vi "Dashboard Main.vi"() -> ()   [LabVIEW 2013]
uses:
  <vilib>/event_ctls.llb/eventvkey.ctl
  <vilib>/Rock Robotics/WPI/Dashboard/WPI_DashboardLogging Global.vi
  <vilib>/Utility/config.llb/Write Key (String).vi
  <vilib>/Utility/config.llb/Write Key (I32).vi
  <vilib>/Utility/config.llb/NI_LVConfig.lvlib
panel:
  out "Image Message":string="Timeout in Camera Communications"
  in  "Rec Mode":enum32{"Stop", "Record", "Playback"}(radio)
  in  "Dashboard Tab":T1(tab)
  out "Pressure":dbl
  out "?":bool
  in  "?":bool
  out "Shoot":bool
  out "Rear Right Power":dbl(slide) scale=0.0..1.0
  out "Front Right Power":dbl(slide) scale=0.0..1.0
  out "Front Left Power":dbl(slide) scale=0.0..1.0
  out "Front Left Wheel":dbl(knob) scale=-3.14..3.14
  out "Front Right Wheel":dbl(knob) scale=-3.14..3.14
  out "Rear Right Wheel":dbl(knob) scale=-3.14..3.14
  in  "Camera Settings":T2={"Frame Rate"=30, "Compression"=30, "Size"=1} {"Frame Rate" scale=1.0..30.0; "Size" items=["640x480", "320x240", "160x120"]}
  out "Mode":T3(ring)=enum."Auto Disabled"
  out "Camera IP":string
  in  "DB Camera Config":bool
  out "fps":dbl format="%#.1g"
  out "Mbps":dbl format="%#.1g"
  out "Mbps 2":bool
  out "Rear Left Wheel":dbl(knob) scale=-3.14..3.14
  out "Rear Left Power":dbl(slide) scale=0.0..1.0
  in  "Slider 1":dbl(slide) scale=0.0..100.0
  in  "Autonomous Type":u16(ring) items=["One Ball", "Two Ball", "Basic"]
  in  "Test Slider":dbl(slide) scale=0.0..100.0 scale format="%#_3g"
  in  "On/Off":bool caption="Solenoid"
  in  "Test Name":u16(ring) items=["Select the test to run...", "Example Test", "-------------------------------", "List of tests is built in robot code.", "Replace with your own automated tests."]
  in  "Test Tree":string(tree)
  in  "Motor":cluster{"Value":dbl, "Enable":bool} {"Value" scale=-1.0..1.0 scale format="%#_3g"}
  out "Progress":T4 {"Test Progress" scale=0.0..100.0}
  in  "Rev/Fwd":cluster{"Forward":bool, "Reverse":bool}
  in  "Test Ring":u16(ring) items=["Auto", "Fixed indoor", "Fixed outdoor 1", "Fixed outdoor 2", "Fixed fluorescent 1", "Fixed fluorescent 2", "Hold current"]
  in  "Listbox":i32(listbox)
  out "Tree":string(tree)
  out "Camera Image":T5(plugin-control)
  in  "Enable":bool
  # "Customize by placing controls and indicators here and name to\nmatch Dashboard Variables on robot."
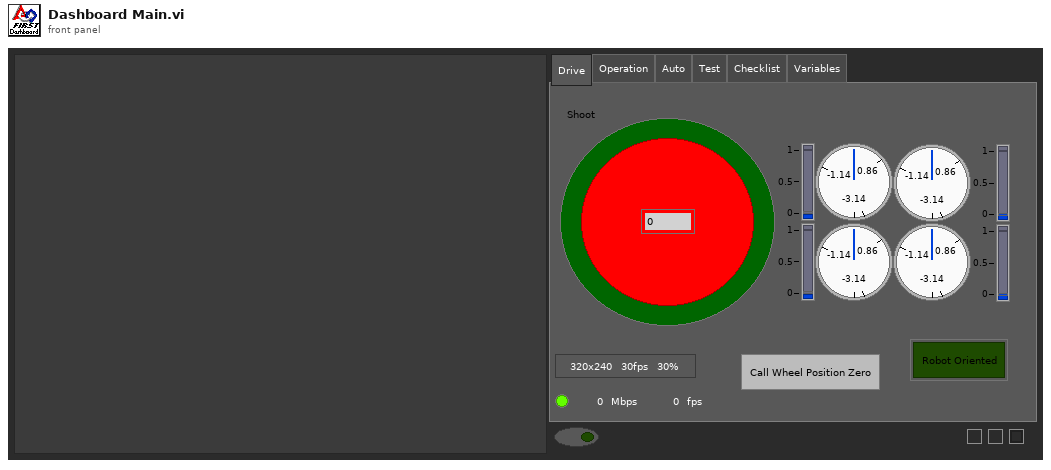
[diagram p1: front panel]
types:
  T1 = enum32{"Drive", "Operation", "Auto", "Test", "Checklist", "Variables"}
  T2 = cluster{"Frame Rate":i32, "Compression":i32, "Size":u16}
  T3 = enum8{"Tele-Op Disabled", "Tele-Op Enabled", "Auto Disabled", "Auto Enabled", "Test Disabled", "Test Enabled", ""}
  T4 = cluster{"Test Progress":u8, "Test Progress Text":string}
  T5 = typedef "IMAQ Image.ctl" = refnum<image>
  T6 = typedef "Image Type" = u32
  T7 = cluster{"Digital Inputs":bool[], "Digital Outputs":bool[]}
  T8 = cluster{"Competition mode":bool, "Robot Link":bool, "Autonomous":bool, "Enabled":bool, "E-Stop":bool, "Simulated":bool, "TestMode":bool, "Docked Window":bool}
  T9 = typedef "NI_LVConfig.lvlib/Config Data RefNum.ctl" = refnum<k1>
  T10 = typedef "eventvkey.ctl" = enum16{"ASCII", "Enter", "Return", "Shift", "Ctrl", "Alt", "Cmd", "Opt", "Caps", "NumLock", "Clear", "Break", "Up", "Down", "Left", "Right", "Insert", "Delete", "Home", "End", "PageUp", "PageDown", "Escape", "Help", "Pause", "ScrollLock", "F1", "F2", "F3", "F4", "F5", "F6", "F7", "F8", "F9", "F10", "F11", "F12", "F13", "F14", "F15", "F16", "F17", "F18", "F19", "F20", "F21", "F22", "F23", "F24", "Play", "VolumeUp", "VolumeDown", "Mute", "Two Byte Char"}
  T11 = cluster{"Image Size":bool, "Image Type":bool, "Pixel Value":bool, "ROI Information":bool, "Zoom Factor":bool}
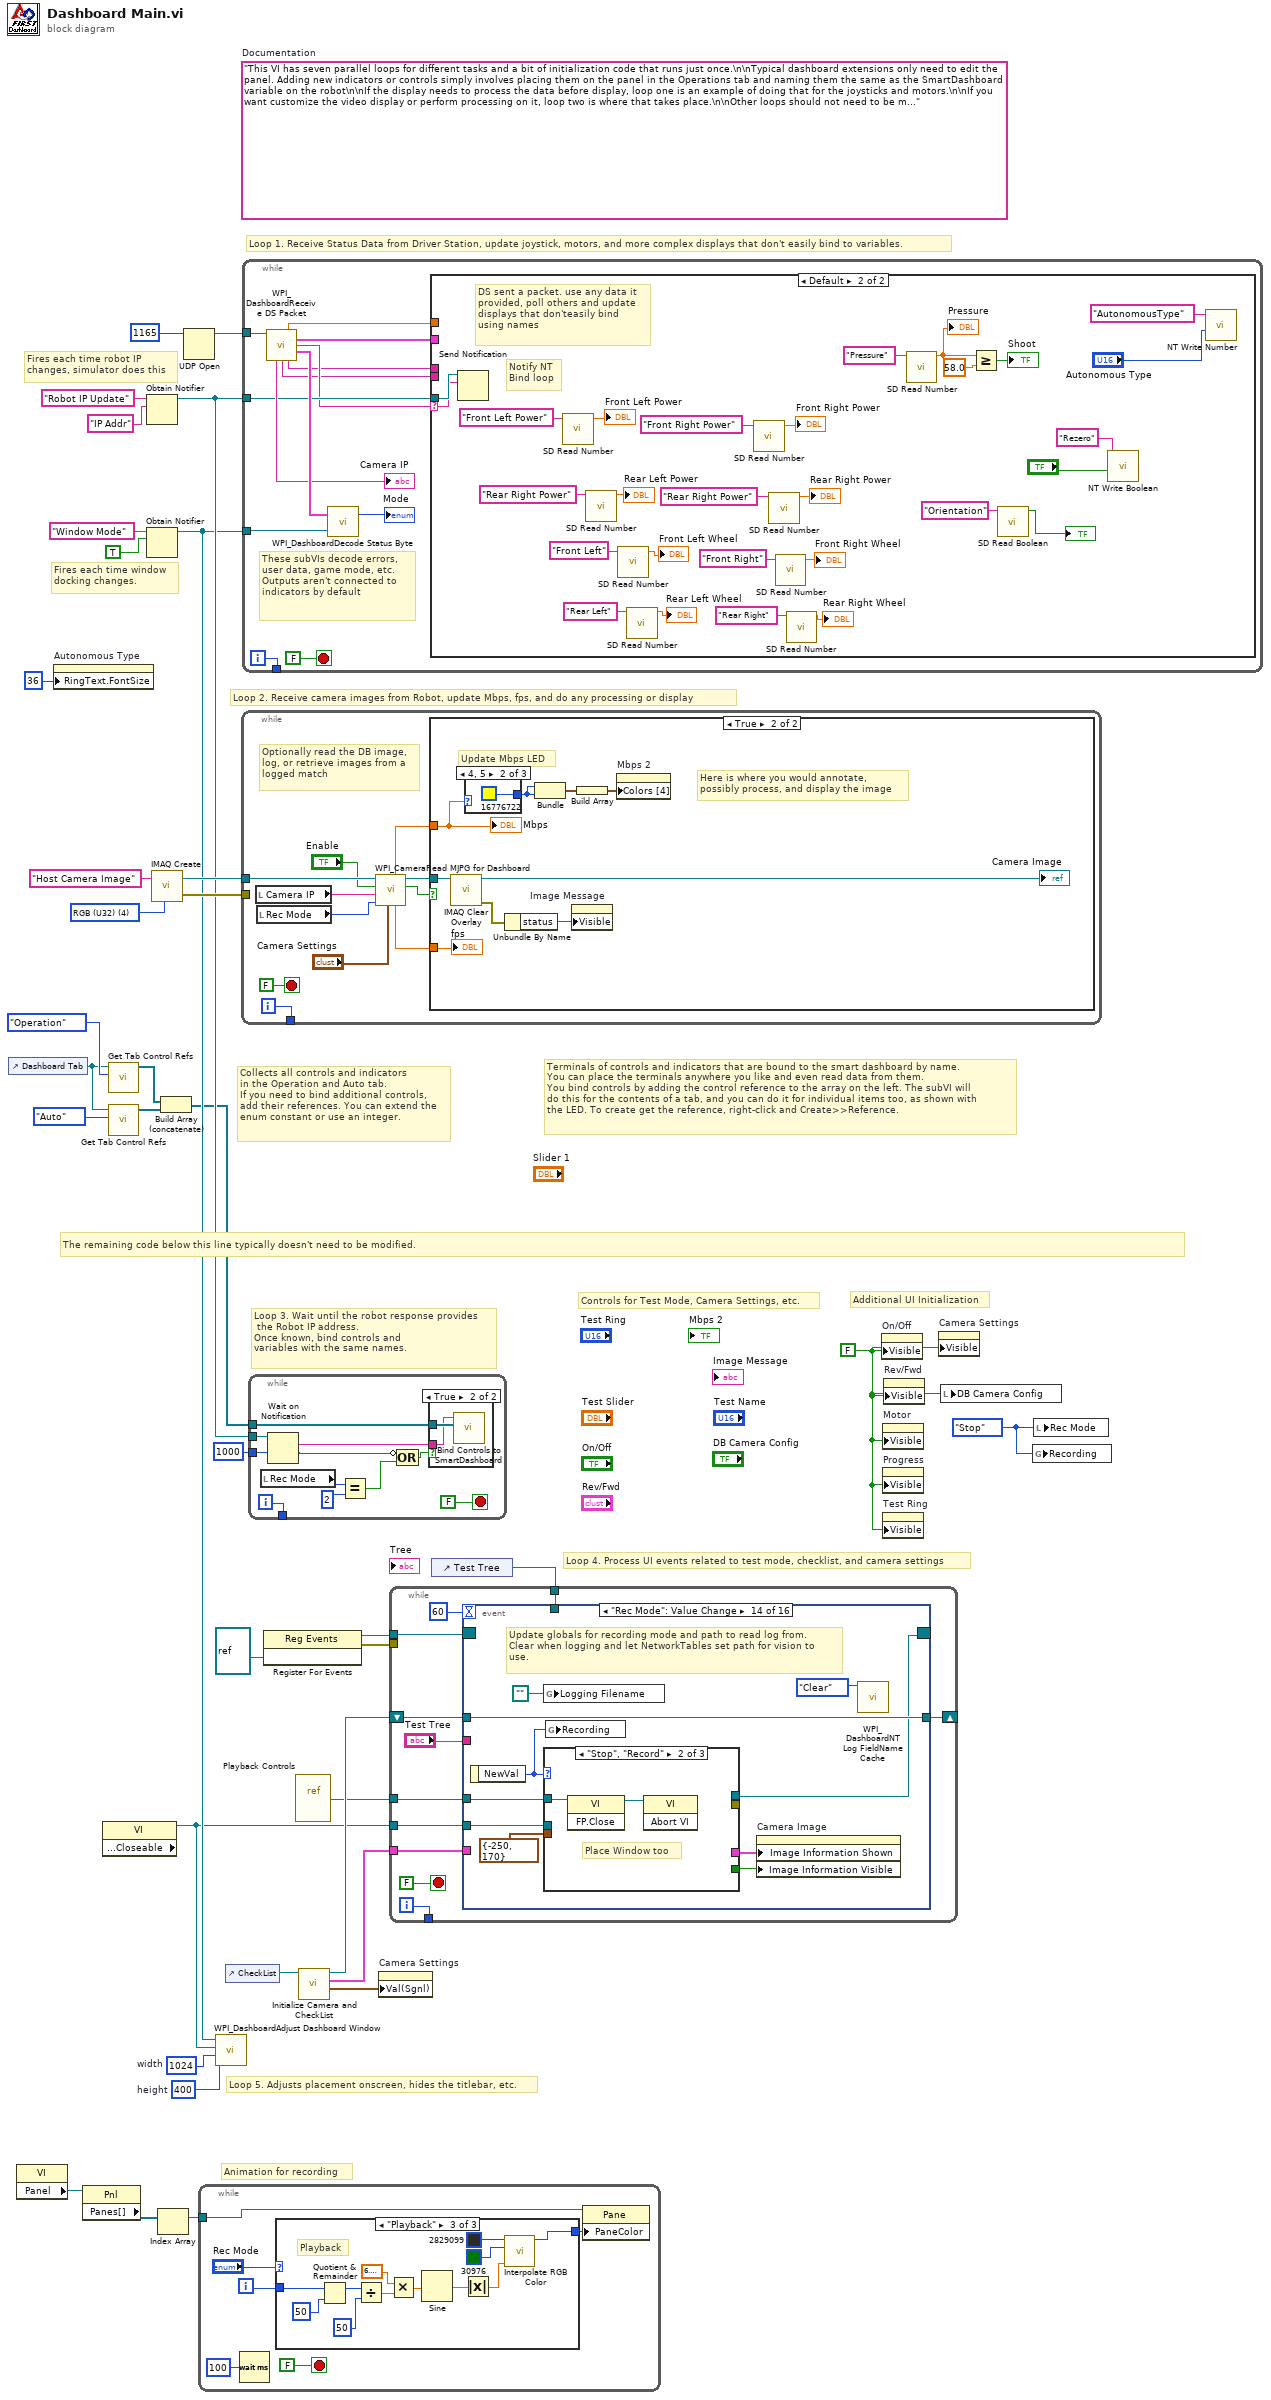
[diagram p0: block diagram]
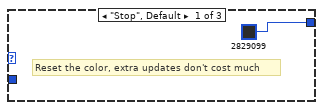
[diagram p2: hidden frame]
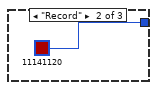
[diagram p3: hidden frame]
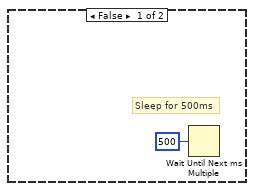
[diagram p5: hidden frame]
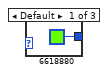
[diagram p6: hidden frame]
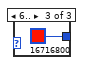
[diagram p7: hidden frame]
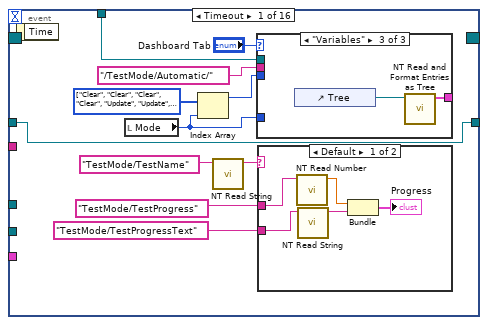
[diagram p8: hidden frame]
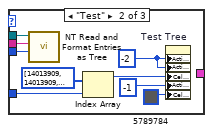
[diagram p10: hidden frame]
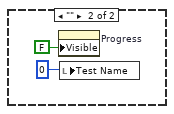
[diagram p11: hidden frame]
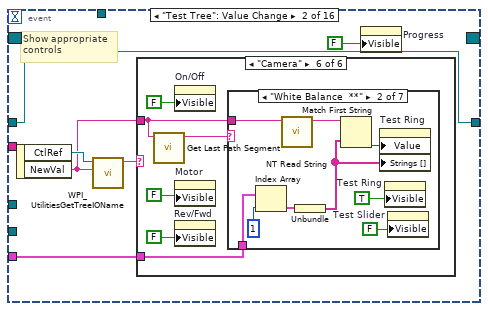
[diagram p12: hidden frame]
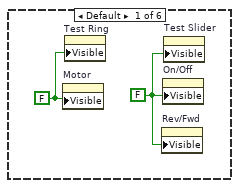
[diagram p13: hidden frame]
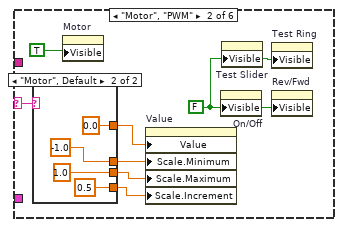
[diagram p14: hidden frame]
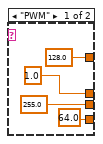
[diagram p15: hidden frame]
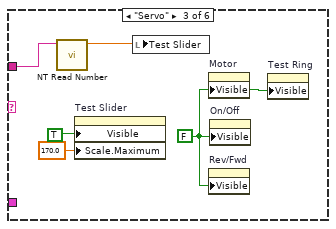
[diagram p16: hidden frame]
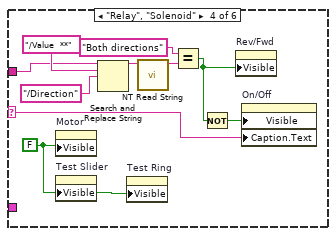
[diagram p17: hidden frame]
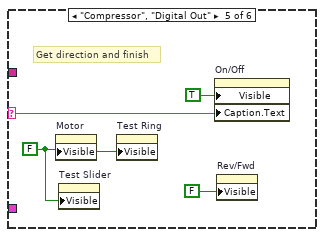
[diagram p18: hidden frame]
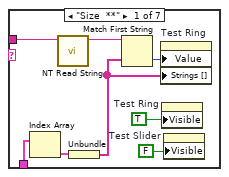
[diagram p19: hidden frame]
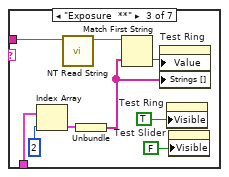
[diagram p20: hidden frame]
diagram:
  w8 = enum32{"Stop", "Record", "Playback"}."Stop" ("Rec Mode")
  w11 = 400  # height
  w12 = 1024  # width
  w25 = FALSE ("Visible")
  (unwired) "This VI has seven parallel loops for different tasks and a bit of initialization code that runs just once.\n\nTypical dashboard extensions only need to edit the panel. Adding new indicators or controls simply involves placing them on the panel in the Operations tab and naming them the same as the SmartDashboard variable on the robot\n\nIf the display needs to process the data before display, loop one is an example of doing that for the joysticks and motors.\n\nIf you want customize the video display or perform processing on it, loop two is where that takes place.\n\nOther loops should not need to be modified. They are pretty standard, and document the task they perform."  # Documentation
  w35 = T6 4 items=["Grayscale (U8)", "Grayscale (I16)", "Grayscale (SGL)", "Complex (CSG)", "RGB (U32)", "HSL (U32)", "RGB (U64)"] ("Image Type")
  # "Controls for Test Mode, Camera Settings, etc."
  # "Additional UI Initialization"
  # "Animation for recording"
  # "Fires each time robot IP\nchanges, simulator does this"
  # "Fires each time window\ndocking changes."
  # "Collects all controls and indicators\nin the Operation and Auto tab.\nIf you need to bind additional controls,\nadd their references. You can extend the\nenum constant or use an integer."
  # "The remaining code below this line typically doesn't need to be modified."
  # "Loop 4. Process UI events related to test mode, checklist, and camera settings"
  # "Terminals of controls and indicators that are bound to the smart dashboard by name.\nYou can place the terminals anywhere you like and even read data from them.\nYou bind controls by adding the control reference to the array on the left. The subVI will\ndo this for the contents of a tab, and you can do it for individual items too, as shown with\nthe LED. To create get the reference, right-click and Create>>Reference."
  # "Loop 3. Wait until the robot response provides\n the Robot IP address.\nOnce known, bind controls and\nvariables with the same names."
  # "Loop 5. Adjusts placement onscreen, hides the titlebar, etc."
  # "Loop 1. Receive Status Data from Driver Station, update joystick, motors, and more complex displays that don't easily bind to variables."
  # "Loop 2. Receive camera images from Robot, update Mbps, fps, and do any processing or display"
  n1 = control-ref of="Dashboard Tab"() -> (w6:refnum<vi>)
  n2 = property class="VI"() -> ("Panel"=w19:refnum<vi>)  [unwired: 2 in, 2 out]
  n3 = property on="Autonomous Type" class="Ring (strict)"("RingText.FontSize"=u32 36 ("Ring Text.Font:Size")) -> ()  [unwired: 2 in, 2 out]
  n4 = property class="Pnl"(reference=w19) -> ("Panes[]"=w20:refnum<vi>[])  [unwired: 1 in, 2 out]
  n5 = property class="VI" props=["Front Panel.Closeable"]() -> (reference out=w7:refnum<vi>)  [unwired: 2 in, 2 out]
  n6 = call <vilib>:"Get Tab Control Refs.vi"("Page Index"=T1."Operation" ("Dashboard Tab"), "TabControl in"=w6) -> ("ControlsOnPage"=w4:refnum<vi>[])  [unwired: 9 in]
  n7 = call <vilib>:"Get Tab Control Refs.vi"("Page Index"=T1."Auto" ("Dashboard Tab"), "TabControl in"=w6) -> ("ControlsOnPage"=w5:refnum<vi>[])  [unwired: 9 in]
  n8 = Obtain Notifier(name (unnamed)="Robot IP Update", notification data type="IP Addr" ("name (unnamed)")) -> (notifier out=w29:refnum<notifier>)  [unwired: 2 in, 2 out]
  n9 = Obtain Notifier(name (unnamed)="Window Mode", notification data type=TRUE) -> (notifier out=w10:refnum<notifier>)  [unwired: 2 in, 2 out]
  n10 = call "IMAQ Create"("Image Name"="Host Camera Image", "Image Type"=w35) -> ("New Image"=w33:T5, "error out"=w32:errorcluster)  [unwired: 2 in, 1 out]
  n11 = Index Array(array=w20) -> (element=w18:refnum<vi>)  [unwired: 1 in]
  n12 = Build Array (concatenate)(w4, w5) -> (w3:refnum<vi>[])
  n13 = UDP Open(11:u16 1165 ("port")) -> (port=w36:refnum<k16>)  [unwired: 2 in, 4 out]
  n14 = while {
    tunnel: w18 -> [w39]
    i -> [w42]
    stop <- FALSE stop-if-true
    n15 = Wait (ms)(milliseconds to wait=u32 100) -> ()  [unwired: 1 out]
    n16 = case shown="\"Playback\"" "Rec Mode" {
      tunnel: w42 -> [_ _ w57]
      tunnel: [u32 2829099 ("Base Color") u32 11141120 ("Target Color") w46] -> w38
      frame "Stop", Default {
        # "Reset the color, extra updates don't cost much"
      }
      frame "Record" {
      }
      frame "Playback" {
        # "Playback"
        n17 = Quotient & Remainder(x=w57, y=u32 50 ("milliseconds to wait")) -> (x-y*floor(x/y)=w53:u32)  [unwired: 1 out]
        n18 = Divide(x=w53, y=u32 50 ("milliseconds to wait")) -> (x/y=w50:dbl)
        n19 = Multiply(x=6.283185307179586, y=w50) -> (x*y=w55:dbl)
        n20 = Sine(x=w55) -> (sin(x)=w54:dbl)
        n21 = Absolute Value(x=w54) -> (abs(x)=w47:dbl)
        n22 = call "Interpolate RGB Color.vi"("Proportion"=w47, "Target Color"=u32 30976, "Base Color"=u32 2829099) -> ("Result Color"=w46:u32)  [unwired: 8 in]
      }
    }
    n23 = property class="Pane"(reference=w39, "PaneColor"=w38) -> ()  [unwired: 1 in, 2 out]
  }
  n24 = call <vilib>:"WPI_DashboardAdjust Dashboard Window.vi"("height"=w11, "width"=w12, "reference in"=w7, "Notifier in"=w10) -> ()  [unwired: 8 in]
  n25 = control-ref of="CheckList"() -> (w9:refnum<vi>)
  n26 = while {
    tunnel: w33 -> [w66]
    tunnel: w32 -> [_]
    tunnel: [w67] -> _
    i -> [w67]
    stop <- FALSE stop-if-true
    # "Optionally read the DB image,\nlog, or retrieve images from a\nlogged match"
    n27 = local read "Camera IP"() -> (w59:string)
    n28 = local read "Rec Mode"() -> (w58:enum32{"Stop", "Record", "Playback"})
    n29 = call <vilib>:"WPI_CameraRead MJPG for Dashboard.vi"("Camera Settings"="Camera Settings", "Rec Mode"=w58, "Camera IP"=w59, "Enable"="Enable", "Refnum in"=w66) -> ("Active"=w63:bool, "Refnum out"=w65:T5, "FPS"=w62:dbl, "Bandwidth (Mbps)"=w61:dbl)  [unwired: 3 in]
    n30 = case shown="True" w63 {
      tunnel: w65 -> [_ w73]
      tunnel: w61 -> [_ w72]
      tunnel: w62 -> [_ w70]
      frame False {
        # "Sleep for 500ms"
        n31 = Wait Until Next ms Multiple(millisecond multiple=u32 500) -> ()  [unwired: 1 out]
      }
      frame True {
        # "Here is where you would annotate,\npossibly process, and display the image"
        # "Update Mbps LED"
        n32 = call "IMAQ Clear Overlay"("Image"=w73) -> ("error out"=w77:errorcluster, "Image Out"=→"Camera Image":T5)  [unwired: 2 in, 7 out]
        n33 = case shown="4, 5" w72 {
          tunnel: [u32 6618880 ("Color Box") u32 16776722 ("Color Box") u32 16716800 ("Color Box")] -> w74
          frame Default {
          }
          frame 4, 5 {
          }
          frame 6.. {
          }
        }
        n34 = Unbundle By Name(w77) -> ("status"=w78:bool)
        n35 = Bundle("Color Box"=w74, "Color Box"=w74) -> (w76:cluster{"Color Box":u32, "Color Box":u32})  [unwired: 1 out]
        n36 = property on="Image Message" class="Str"("Visible"=w78) -> ()  [unwired: 2 in, 2 out]
        n37 = Build Array(w76) -> (w75:cluster{"Color Box":u32, "Color Box":u32}[])
        n38 = property on="Mbps 2" class="Bool (strict)"("Colors [4]"=w75) -> ()  [unwired: 2 in, 2 out]
        "Mbps" <- w72
        "fps" <- w70
      }
    }
  }
  n39 = while {
    tunnel: w36 -> [w92]
    tunnel: w29 -> [w87]
    tunnel: w10 -> [w91]
    tunnel: [w88] -> _
    i -> [w88]
    stop <- FALSE stop-if-true
    # "These subVIs decode errors, user data, game mode, etc.\nOutputs aren't connected to indicators by default"
    n40 = call <vilib>:"WPI_DashboardReceive DS Packet.vi"("Recv Socket"=w92) -> ("Battery"=w82:sgl, "Driver Station"=w83:T7, "Robot IP Address"=w86:string, "Status"=w93:T8, "Camera IP Address"=→"Camera IP":string, "Low Priority User Data"=w85:string, "High Priority User Data"=w84:string)  [unwired: 1 in, 7 out]
    n41 = call <vilib>:"WPI_DashboardDecode Status Byte.vi"("Window Mode Notifier"=w91, "Status"=w93) -> ("Mode"=→"Mode":T3)  [unwired: 1 out]
    n42 = case shown="Default" w86 {
      selector: w86 -> [_ w121]
      tunnel: w87 -> [_ w122]
      tunnel: w85 -> [_ _]
      tunnel: w84 -> [_ _]
      tunnel: w83 -> [_ _]
      tunnel: w82 -> [_ _]
      frame "0.0.0.0" {
        # "DS not sending packets, or no robot exists yet.\nDon't poll the variables"
      }
      frame Default {
        # "Notify NT\nBind loop"
        # "DS sent a packet. use any data it\nprovided, poll others and update\ndisplays that don'teasily bind\nusing names"
        n43 = Send Notification(notification=w121, notifier=w122) -> ()  [unwired: 1 in, 2 out]
        n44 = call <vilib>:"SD Read Number.vi"("Name"="Front Left Power") -> ("Numeric"=→"Front Left Power":dbl)  [unwired: 8 in, 2 out]
        n45 = call <vilib>:"SD Read Number.vi"("Name"="Rear Right Power") -> ("Numeric"=→"Rear Left Power":dbl)  [unwired: 8 in, 2 out]
        n46 = call <vilib>:"SD Read Number.vi"("Name"="Front Left") -> ("Numeric"=→"Front Left Wheel":dbl)  [unwired: 8 in, 2 out]
        n47 = call <vilib>:"SD Read Number.vi"("Name"="Rear Left") -> ("Numeric"=→"Rear Left Wheel":dbl)  [unwired: 8 in, 2 out]
        n48 = call <vilib>:"SD Read Number.vi"("Name"="Front Right Power") -> ("Numeric"=→"Front Right Power":dbl)  [unwired: 8 in, 2 out]
        n49 = call <vilib>:"SD Read Number.vi"("Name"="Rear Right Power") -> ("Numeric"=→"Rear Right Power":dbl)  [unwired: 8 in, 2 out]
        n50 = call <vilib>:"SD Read Number.vi"("Name"="Front Right") -> ("Numeric"=→"Front Right Wheel":dbl)  [unwired: 8 in, 2 out]
        n51 = call <vilib>:"SD Read Number.vi"("Name"="Rear Right") -> ("Numeric"=→"Rear Right Wheel":dbl)  [unwired: 8 in, 2 out]
        n52 = call <vilib>:"SD Read Number.vi"("Name"="Pressure") -> ("Numeric"=w97:dbl)  [unwired: 8 in, 2 out]
        "Pressure" <- w97
        n53 = Greater Or Equal?(x=w97, y=58.0) -> (x >= y?=→"Shoot":bool)
        n54 = call <vilib>:"SD Read Boolean.vi"("Name"="Orientation") -> ("Boolean"=→"?":bool)  [unwired: 8 in, 2 out]
        n55 = call <vilib>:"NT Write Boolean.vi"("Boolean"="?", "Name"="Rezero") -> ()  [unwired: 9 in, 1 out]
        n56 = call <vilib>:"NT Write Number.vi"("Numeric"="Autonomous Type", "Name"="AutonomousType") -> ()  [unwired: 9 in, 1 out]
      }
    }
  }
  n57 = while {
    tunnel: w3 -> [w133]
    tunnel: w29 -> [w131]
    tunnel: [w129] -> _
    tunnel: u32 1000 ("milliseconds to wait") -> [w128]
    i -> [w129]
    stop <- FALSE stop-if-true
    n58 = local read "Rec Mode"() -> (w124:enum32{"Stop", "Record", "Playback"})
    n59 = Wait on Notification(notifier=w131, timeout in ms (-1)=w128) -> (notification=w130:string, timed out?=w126:bool)  [unwired: 2 in, 2 out]
    n60 = Equal?(x=w124, y=u16 2 ("Rec Mode")) -> (x = y?=w125:bool)
    n61 = Compound Arithmetic op=OR(invert w126, w125) -> (w127:bool)
    n62 = case shown="True" w127 {
      tunnel: w133 -> [_ w135]
      tunnel: w130 -> [_ w134]
      frame False {
      }
      frame True {
        n63 = call <vilib>:"Bind Controls to SmartDashboard.vi"("Bound Control Refs"=w135, "Server IP Address"=w134) -> ()  [unwired: 10 in]
      }
    }
  }
  n64 = register-events(refnum<vi> refnum) -> (reference out=w16:refnum<event-registration>, error out=w15:errorcluster)  [unwired: 2 in]
  n65 = vi-ref "Playback Controls.vi"() -> (w17:refnum<vi>)
  n66 = call "Initialize Camera and CheckList.vi"("ListBox in"=w9) -> ("Cluster"=w23:cluster{"value":i32, "value":i32, "index":i32}, "Array"=w24:cluster{string[]}[], "File Refnum"=w22:T9)  [unwired: 8 in]
  n67 = property on="Camera Settings" class="Clust (strict)"("Val(Sgnl)"=w23) -> ()  [unwired: 2 in, 2 out]
  n68 = control-ref of="Test Tree"() -> (w21:refnum<vi>)
  n69 = while {
    tunnel: w24 -> [w143]
    shift-right: [w142] -> _
    shift-left: w22 -> [w141]
    tunnel: [w140] -> _
    tunnel: w21 -> [w139]
    tunnel: w17 -> [w138]
    tunnel: w16 -> [w137]
    tunnel: w15 -> [_]
    tunnel: w7 -> [w136]
    i -> [w140]
    stop <- FALSE stop-if-true
    n70 = event shown="[13] \"Rec Mode\": Value Change" {
      selector: w137 -> [_ _ _ _ _ _ _ _ _ _ _ _ _ _ _ _]
      dyn-events: [_ _ _ _ _ _ _ _ _ _ _ _ _ w381 _ _] -> _
      timeout: u32 60 ("milliseconds to wait") -> [_ _ _ _ _ _ _ _ _ _ _ _ _ _ _ _]
      tunnel: w139 -> [w153 _ _ _ _ _ _ _ _ _ _ _ _ _ _ _]
      tunnel: "Test Tree" -> [_ _ _ _ _ _ _ _ w350 w358 w360 w364 w372 _ _ _]
      tunnel: w143 -> [_ w177 _ _ _ _ w314 w344 _ _ _ _ _ _ _ _]
      tunnel: [w147 w176 w275 w280 w288 w300 w313 w337 w349 w356 w359 w363 w371 w383 w397 w398] -> w142
      tunnel: w141 -> [w147 w176 w275 w280 w288 w300 w312 w337 w349 w356 w359 w363 w371 w383 w397 w398]
      tunnel: w138 -> [_ _ _ _ _ _ _ _ _ _ _ _ _ w384 _ w401]
      tunnel: w136 -> [_ _ _ _ _ _ _ _ _ _ _ _ _ w379 _ _]
      event Timeout {
        w152 = enum16{"Update", "Clear"}[] [enum."Clear", enum."Clear", enum."Clear", enum."Clear", enum."Update", enum."Update", enum."Clear"] items=["Update", "Clear"]
        n71 = event-data() -> ()  [unwired: 1 in, 1 out]
        n72 = local read "Mode"() -> (w150:T3)
        n73 = Index Array(array=w152, index=w150) -> (element=w151:enum16{"Update", "Clear"})
        n74 = call <vilib>:"NT Read String.vi"("Name"="TestMode/TestName") -> ("String"=w156:string)  [unwired: 9 in, 1 out]
        n75 = case shown="\"Variables\"" "Dashboard Tab" {
          tunnel: w153 -> [_ w166 _]
          tunnel: "/TestMode/Automatic/" ("Name Pattern") -> [_ w165 _]
          tunnel: w151 -> [_ w164 _]
          tunnel: w150 -> [_ w162 _]
          tunnel: [_ _ w168] -> _
          frame "Operation", Default {
          }
          frame "Test" {
            w161 = -2 ("Active Item:Row Number")
            n76 = call <vilib>:"NT Read and Format Entries as Tree.vi"("Operation"=w164, "Name Pattern"=w165, "Tree Refnum"=w166) -> ()  [unwired: 7 in, 2 out]
            n77 = Index Array(array=u32[] [14013909, 14013909, 14013909, 14013909, 14013909, 16777215, 14013909], index=w162) -> (element=w160:u32)
            n78 = property on="Test Tree" class="Tree (strict)"("Active Item Row Number"=w161, "ActiveColNum"=w161, "CellBG"=w160, "Active Item Row Number"=-1 ("Active Item:Row Number"), "CellBG"=u32 5789784 ("Color Box")) -> ()  [unwired: 2 in, 2 out]
          }
          frame "Variables" {
            n79 = control-ref of="Tree"() -> (w167:refnum<vi>)
            n80 = call <vilib>:"NT Read and Format Entries as Tree.vi"("Tree Refnum"=w167) -> ("Formatted Strings"=w168:cluster{"Name":string, "Value":string}[])  [unwired: 9 in, 1 out]
          }
        }
        n81 = case shown="Default" w156 {
          tunnel: "TestMode/TestProgress" ("Name") -> [w170 _]
          tunnel: "TestMode/TestProgressText" ("Name") -> [w169 _]
          frame Default {
            n82 = call <vilib>:"NT Read Number.vi"("Name"=w170) -> ("Numeric"=w171:dbl)  [unwired: 9 in, 1 out]
            n83 = call <vilib>:"NT Read String.vi"("Name"=w169) -> ("String"=w172:string)  [unwired: 9 in, 1 out]
            n84 = Bundle("Numeric"=w171, "String"=w172) -> (→"Progress":cluster{"Numeric":dbl, "String":string})  [unwired: 1 in]
          }
          frame "" {
            n85 = property on="Progress" class="Clust (strict)"("Visible"=FALSE) -> ()  [unwired: 2 in, 2 out]
            n86 = local write "Test Name"(u16 0) -> ()
          }
        }
      }
      event "Test Tree": Value Change {
        # "Show appropriate\ncontrols"
        n87 = event-data() -> ("CtlRef"=w180:refnum<vi>, "NewVal"=w178:string)  [unwired: 1 in]
        n88 = call <vilib>:"WPI_UtilitiesGetTreeIOName.vi"("NewVal"=w178, "TreeControl in"=w180) -> ("I/O Name"=w181:string)  [unwired: 9 in]
        n89 = case shown="\"Camera\"" w181 {
          selector: w181 -> [_ w188 _ w206 w215 _]
          tunnel: w178 -> [_ _ w203 w205 _ w222]
          tunnel: w177 -> [_ _ _ _ _ w221]
          frame Default {
            w183 = FALSE ("Visible")
            w182 = FALSE ("Visible")
            n90 = property on="Motor" class="Clust (strict)"("Visible"=w182) -> ()  [unwired: 2 in, 2 out]
            n91 = property on="Test Ring" class="Ring (strict)"("Visible"=w182) -> ()  [unwired: 2 in, 2 out]
            n92 = property on="Rev/Fwd" class="Clust (strict)"("Visible"=w183) -> ()  [unwired: 2 in, 2 out]
            n93 = property on="On/Off" class="Bool (strict)"("Visible"=w183) -> ()  [unwired: 2 in, 2 out]
            n94 = property on="Test Slider" class="Slide (strict)"("Visible"=w183) -> ()  [unwired: 2 in, 2 out]
          }
          frame "Motor", "PWM" {
            w189 = FALSE ("Visible")
            n95 = case shown="\"Motor\", Default" w188 {
              tunnel: [1.0 ("Value") -1.0 ("Value")] -> w187
              tunnel: [255.0 ("Value") 1.0 ("Value")] -> w186
              tunnel: [128.0 ("Value") 0.0 ("Value")] -> w185
              tunnel: [64.0 ("Value") 0.5 ("Value")] -> w184
              frame "PWM" {
              }
              frame "Motor", Default {
              }
            }
            n96 = property on="Motor" class="Clust (strict)"("Visible"=TRUE) -> ()  [unwired: 2 in, 2 out]
            n97 = property on="Value" class="Slide (strict)"("Value"=w185, "Scale.Minimum"=w187, "Scale.Maximum"=w186, "Scale.Increment"=w184) -> ()  [unwired: 2 in, 2 out]
            n98 = property on="On/Off" class="Bool (strict)"("Visible"=w189) -> ()  [unwired: 2 in, 2 out]
            n99 = property on="Test Slider" class="Slide (strict)"("Visible"=w189) -> ()  [unwired: 2 in, 2 out]
            n100 = property on="Test Ring" class="Ring (strict)"("Visible"=w189) -> ()  [unwired: 2 in, 2 out]
            n101 = property on="Rev/Fwd" class="Clust (strict)"("Visible"=w189) -> ()  [unwired: 2 in, 2 out]
          }
          frame "Servo" {
            w201 = FALSE ("Visible")
            n102 = call <vilib>:"NT Read Number.vi"("Name"=w203) -> ("Numeric"=w202:dbl)  [unwired: 9 in, 1 out]
            n103 = property on="Test Slider" class="Slide (strict)"("Visible"=TRUE, "Scale.Maximum"=170.0 ("Scale.Range:Maximum")) -> ()  [unwired: 2 in, 2 out]
            n104 = local write "Test Slider"(w202) -> ()
            n105 = property on="Motor" class="Clust (strict)"("Visible"=w201) -> ()  [unwired: 2 in, 2 out]
            n106 = property on="Rev/Fwd" class="Clust (strict)"("Visible"=w201) -> ()  [unwired: 2 in, 2 out]
            n107 = property on="On/Off" class="Bool (strict)"("Visible"=w201) -> ()  [unwired: 2 in, 2 out]
            n108 = property on="Test Ring" class="Ring (strict)"("Visible"=w201) -> ()  [unwired: 2 in, 2 out]
          }
          frame "Relay", "Solenoid" {
            w204 = FALSE ("Visible")
            n109 = property on="Motor" class="Clust (strict)"("Visible"=w204) -> ()  [unwired: 2 in, 2 out]
            n110 = property on="Test Slider" class="Slide (strict)"("Visible"=w204) -> ()  [unwired: 2 in, 2 out]
            n111 = Search and Replace String(input string=w205, search string="/Value  **", replace string="/Direction") -> (result string=w211:string)  [unwired: 5 in, 3 out]
            n112 = property on="Test Ring" class="Ring (strict)"("Visible"=w204) -> ()  [unwired: 2 in, 2 out]
            n113 = call <vilib>:"NT Read String.vi"("Name"=w211) -> ("String"=w209:string)  [unwired: 9 in, 1 out]
            n114 = Equal?(x="Both directions", y=w209) -> (x = y?=w207:bool)
            n115 = Not(x=w207) -> (.not. x?=w208:bool)
            n116 = property on="Rev/Fwd" class="Clust (strict)"("Visible"=w207) -> ()  [unwired: 2 in, 2 out]
            n117 = property on="On/Off" class="Bool (strict)"("Visible"=w208, "Caption.Text"=w206) -> ()  [unwired: 2 in, 2 out]
          }
          frame "Compressor", "Digital Out" {
            w214 = FALSE ("Visible")
            # "Get direction and finish"
            n118 = property on="Motor" class="Clust (strict)"("Visible"=w214) -> ()  [unwired: 2 in, 2 out]
            n119 = property on="Test Slider" class="Slide (strict)"("Visible"=w214) -> ()  [unwired: 2 in, 2 out]
            n120 = property on="Test Ring" class="Ring (strict)"("Visible"=w214) -> ()  [unwired: 2 in, 2 out]
            n121 = property on="On/Off" class="Bool (strict)"("Visible"=TRUE, "Caption.Text"=w215) -> ()  [unwired: 2 in, 2 out]
            n122 = property on="Rev/Fwd" class="Clust (strict)"("Visible"=FALSE) -> ()  [unwired: 2 in, 2 out]
          }
          frame "Camera" {
            n123 = call <vilib>:"Get Last Path Segment.vi"("String in"=w222) -> ("String out"=w223:string)  [unwired: 10 in]
            n124 = property on="On/Off" class="Bool (strict)"("Visible"=FALSE) -> ()  [unwired: 2 in, 2 out]
            n125 = property on="Motor" class="Clust (strict)"("Visible"=FALSE) -> ()  [unwired: 2 in, 2 out]
            n126 = property on="Rev/Fwd" class="Clust (strict)"("Visible"=FALSE) -> ()  [unwired: 2 in, 2 out]
            n127 = case shown="\"White Balance  **\"" w223 {
              tunnel: w222 -> [w229 w238 w247 w256 w265 _ w271]
              tunnel: w221 -> [w227 w235 w244 w253 w262 _ _]
              frame "Size  **" {
                n128 = Index Array(array=w227) -> (element=w226:cluster{string[]})  [unwired: 1 in]
                n129 = call <vilib>:"NT Read String.vi"("Name"=w229) -> ("String"=w228:string)  [unwired: 9 in, 1 out]
                n130 = Unbundle(w226) -> (w224:string[])
                n131 = Match First String(2:w224, 3:w228) -> (0:w225:i32)  [unwired: 1 out]
                n132 = property on="Test Ring" class="Ring (strict)"("Value"=w225, "Strings []"=w224) -> ()  [unwired: 2 in, 2 out]
                n133 = property on="Test Ring" class="Ring (strict)"("Visible"=TRUE) -> ()  [unwired: 2 in, 2 out]
                n134 = property on="Test Slider" class="Slide (strict)"("Visible"=FALSE) -> ()  [unwired: 2 in, 2 out]
              }
              frame "White Balance  **" {
                n135 = Index Array(array=w235, index=1) -> (element=w236:cluster{string[]})
                n136 = call <vilib>:"NT Read String.vi"("Name"=w238) -> ("String"=w237:string)  [unwired: 9 in, 1 out]
                n137 = Unbundle(w236) -> (w233:string[])
                n138 = Match First String(2:w233, 3:w237) -> (0:w232:i32)  [unwired: 1 out]
                n139 = property on="Test Ring" class="Ring (strict)"("Value"=w232, "Strings []"=w233) -> ()  [unwired: 2 in, 2 out]
                n140 = property on="Test Ring" class="Ring (strict)"("Visible"=TRUE) -> ()  [unwired: 2 in, 2 out]
                n141 = property on="Test Slider" class="Slide (strict)"("Visible"=FALSE) -> ()  [unwired: 2 in, 2 out]
              }
              frame "Exposure  **" {
                n142 = Index Array(array=w244, index=2) -> (element=w245:cluster{string[]})
                n143 = call <vilib>:"NT Read String.vi"("Name"=w247) -> ("String"=w246:string)  [unwired: 9 in, 1 out]
                n144 = Unbundle(w245) -> (w241:string[])
                n145 = Match First String(2:w241, 3:w246) -> (0:w242:i32)  [unwired: 1 out]
                n146 = property on="Test Ring" class="Ring (strict)"("Value"=w242, "Strings []"=w241) -> ()  [unwired: 2 in, 2 out]
                n147 = property on="Test Ring" class="Ring (strict)"("Visible"=TRUE) -> ()  [unwired: 2 in, 2 out]
                n148 = property on="Test Slider" class="Slide (strict)"("Visible"=FALSE) -> ()  [unwired: 2 in, 2 out]
              }
              frame "Exposure Priority  **" {
                n149 = Index Array(array=w253, index=3) -> (element=w254:cluster{string[]})
                n150 = call <vilib>:"NT Read String.vi"("Name"=w256) -> ("String"=w255:string)  [unwired: 9 in, 1 out]
                n151 = Unbundle(w254) -> (w250:string[])
                n152 = Match First String(2:w250, 3:w255) -> (0:w251:i32)  [unwired: 1 out]
                n153 = property on="Test Ring" class="Ring (strict)"("Value"=w251, "Strings []"=w250) -> ()  [unwired: 2 in, 2 out]
                n154 = property on="Test Ring" class="Ring (strict)"("Visible"=TRUE) -> ()  [unwired: 2 in, 2 out]
                n155 = property on="Test Slider" class="Slide (strict)"("Visible"=FALSE) -> ()  [unwired: 2 in, 2 out]
              }
              frame "Color Enable  **" {
                n156 = Index Array(array=w262, index=4) -> (element=w263:cluster{string[]})
                n157 = call <vilib>:"NT Read String.vi"("Name"=w265) -> ("String"=w264:string)  [unwired: 9 in, 1 out]
                n158 = Unbundle(w263) -> (w259:string[])
                n159 = Match First String(2:w259, 3:w264) -> (0:w260:i32)  [unwired: 1 out]
                n160 = property on="Test Ring" class="Ring (strict)"("Value"=w260, "Strings []"=w259) -> ()  [unwired: 2 in, 2 out]
                n161 = property on="Test Ring" class="Ring (strict)"("Visible"=TRUE) -> ()  [unwired: 2 in, 2 out]
                n162 = property on="Test Slider" class="Slide (strict)"("Visible"=FALSE) -> ()  [unwired: 2 in, 2 out]
              }
              frame Default {
                n163 = property on="Test Ring" class="Ring (strict)"("Visible"=FALSE) -> ()  [unwired: 2 in, 2 out]
                n164 = property on="Test Slider" class="Slide (strict)"("Visible"=FALSE) -> ()  [unwired: 2 in, 2 out]
              }
              frame "Brightness  **", "Color Level  **", "Compression  **", "FPS  **", "Sharpness  **" {
                n165 = call <vilib>:"NT Read Number.vi"("Name"=w271) -> ("Numeric"=w270:dbl)  [unwired: 9 in, 1 out]
                n166 = local write "Test Slider"(w270) -> ()
                n167 = property on="Test Slider" class="Slide (strict)"("Visible"=TRUE, "Scale.Maximum"=100.0 ("Scale.Range:Maximum")) -> ()  [unwired: 2 in, 2 out]
                n168 = property on="Test Ring" class="Ring (strict)"("Visible"=FALSE) -> ()  [unwired: 2 in, 2 out]
              }
            }
          }
        }
        n169 = property on="Progress" class="Clust (strict)"("Visible"=FALSE) -> ()  [unwired: 2 in, 2 out]
      }
      event "Test Name": Mouse Enter {
        # "Populate the ring with the list of tests"
        n170 = event-data() -> ()  [unwired: 1 in, 1 out]
        n171 = call <vilib>:"NT Read String Array.vi"("Name"="TestMode/TestList") -> ("String Array"=w279:string[])  [unwired: 9 in, 1 out]
        n172 = Build Array (concatenate)("Select the test to run...", w279) -> (w278:string[])
        n173 = property on="Test Name" class="Ring (strict)"("Strings []"=w278) -> ()  [unwired: 2 in, 2 out]
      }
      event "Test Name": Value Change {
        w281 = FALSE ("Visible")
        # "Tell the robot the test name to run"
        n174 = event-data() -> ("NewVal"=w285:u16)  [unwired: 1 in]
        n175 = property on="Test Name" class="Ring (strict)"() -> ("Strings []"=w286:string[])  [unwired: 2 in, 2 out]
        n176 = local write "Progress"(T4 {"Test Progress"=0, "Test Progress Text"=""} ("Progress")) -> ()
        n177 = Index Array(array=w286, index=w285) -> (element=w284:string)
        n178 = call <vilib>:"NT Write String.vi"("String"=w284, "Name"="TestMode/TestName") -> ()  [unwired: 9 in, 1 out]
        n179 = property on="Progress" class="Clust (strict)"("Visible"=TRUE) -> ()  [unwired: 2 in, 2 out]
        n180 = property on="Motor" class="Clust (strict)"("Visible"=w281) -> ()  [unwired: 2 in, 2 out]
        n181 = property on="Test Slider" class="Slide (strict)"("Visible"=w281) -> ()  [unwired: 2 in, 2 out]
        n182 = property on="On/Off" class="Bool (strict)"("Visible"=w281) -> ()  [unwired: 2 in, 2 out]
        n183 = property on="Rev/Fwd" class="Clust (strict)"("Visible"=w281) -> ()  [unwired: 2 in, 2 out]
        n184 = property on="Test Ring" class="Ring (strict)"("Visible"=w281) -> ()  [unwired: 2 in, 2 out]
      }
      event "Listbox": Double Click {
        n185 = event-data() -> ("PlatMods.Shift"=w289:bool, "Row"=w291:i32)  [unwired: 1 in]
        n186 = case shown="True" w289 {
          tunnel: w291 -> [w295 _]
          tunnel: 1 -> [w294 _]
          frame False {
            n187 = property on="Listbox" class="LstBox (strict)"() -> ("Item Symbols"=w293:i32[])  [unwired: 2 in, 2 out]
            n188 = Replace Array Subset(array=w293, new element=w294, index=w295) -> (w292:i32[])
            n189 = property on="Listbox" class="LstBox (strict)"("Item Symbols"=w292) -> ()  [unwired: 2 in, 2 out]
          }
          frame True {
            w296 = 0 ("Top Row")
            n190 = property on="Listbox" class="LstBox (strict)"() -> ("Number of Rows"=w298:u32)  [unwired: 2 in, 2 out]
            n191 = Initialize Array(0, w298) -> (w297:i32[])
            n192 = property on="Listbox" class="LstBox (strict)"("Top Row"=w296, "Value"=w296, "Item Symbols"=w297) -> ()  [unwired: 2 in, 2 out]
          }
        }
      }
      event "Listbox": Key Down {
        n193 = event-data() -> ("VKey"=w302:T10)  [unwired: 1 in]
        n194 = case shown="\"Left\", \"Right\"" w302 {
          selector: w302 -> [w307 _]
          tunnel: eventvkey."Left" ("VKey") -> [w305 _]
          frame "Left", "Right" {
            n195 = Equal?(x=w305, y=w307) -> (x = y?=w306:bool)
            n196 = Select(t=0, s=w306, f=1) -> (s? t:f=w308:i32)
            n197 = property on="Listbox" class="LstBox (strict)"() -> ("Item Symbols"=w311:i32[])  [unwired: 2 in, 2 out]
            n198 = Replace Array Subset(array=w311, new element=w308, index="Listbox") -> (w310:i32[])
            n199 = property on="Listbox" class="LstBox (strict)"("Item Symbols"=w310) -> ()  [unwired: 2 in, 2 out]
          }
          frame Default {
          }
        }
      }
      event "DB Camera Config": Value Change {
        n200 = event-data() -> ("NewVal"=w315:bool)  [unwired: 1 in]
        n201 = case shown="False" w315 {
          tunnel: w314 -> [w324 _]
          tunnel: [w317 w335] -> w313
          tunnel: w312 -> [w316 w335]
          frame False {
            w331 = "Camera"
            w334 = FALSE ("Visible")
            n202 = local read "Camera Settings"() -> (w323:T2)
            n203 = Index Array(array=w324) -> (element=w327:cluster{string[]})  [unwired: 1 in]
            n204 = Unbundle(w323) -> ("Frame Rate"=w322:i32, "Compression"=w321:i32, "Size"=w325:u16)
            n205 = Unbundle(w327) -> (w326:string[])
            n206 = Index Array(array=w326, index=w325) -> (element=w320:string)
            n207 = call-poly <vilib>:"Write Key.vi"("section"=w331, "value"=w320, "key"="Size", "refnum"=w316) -> ("refnum out"=w333:T9)  [unwired: 2 in, 5 out]
            n208 = call-poly <vilib>:"Write Key.vi"("section"=w331, "value"=w322, "key"="FrameRate", "refnum"=w333) -> ("refnum out"=w332:T9)  [unwired: 1 in, 6 out]
            n209 = property on="Camera Settings" class="Clust (strict)"("Visible"=w334) -> ()  [unwired: 2 in, 2 out]
            n210 = local write "DB Camera Config"(w334) -> ()
            n211 = call-poly <vilib>:"Write Key.vi"("section"=w331, "value"=w321, "key"="Compression", "refnum"=w332) -> ("refnum out"=w318:T9)  [unwired: 1 in, 6 out]
            n212 = call <vilib>:"Close Config Data.vi"("refnum"=w318) -> ("file path"=w319:path)  [unwired: 2 in, 8 out]
            n213 = call <vilib>:"Open Config Data.vi"("configuration file path"=w319) -> ("refnum"=w317:T9)  [unwired: 8 in, 2 out]
          }
          frame True {
            n214 = property on="Camera Settings" class="Clust (strict)"("Visible"=TRUE) -> ()  [unwired: 2 in, 2 out]
          }
        }
      }
      event "Camera Settings": Value Change {
        n215 = event-data() -> ("NewVal"=w348:T2)  [unwired: 1 in]
        n216 = Index Array(array=w344) -> (element=w343:cluster{string[]})  [unwired: 1 in]
        n217 = Unbundle(w348) -> ("Frame Rate"=w339:i32, "Compression"=w338:i32, "Size"=w341:u16)
        n218 = Unbundle(w343) -> (w342:string[])
        n219 = Index Array(array=w342, index=w341) -> (element=w340:string)
        n220 = Format Into String(format string="%s   %dfps   %d%%", w340, w339, w338) -> (resulting string=w345:string)  [unwired: 2 in, 1 out]
        n221 = Build Array(w345) -> (w346:string[])
        n222 = property on="DB Camera Config" class="Bool (strict)"("Strings [4]"=w346) -> ()  [unwired: 2 in, 2 out]
      }
      event "Motor.Enable": Value Change {
        n223 = event-data() -> ("NewVal"=w354:bool)  [unwired: 1 in]
        n224 = Unbundle("Motor") -> ("Value"=w353:dbl)  [unwired: 1 out]
        n225 = Select(t=w353, s=w354, f=0.0) -> (s? t:f=w351:dbl)
        n226 = call <vilib>:"NT Write Number.vi"("Numeric"=w351, "Name"=w350) -> ()  [unwired: 9 in, 1 out]
      }
      event "Test Slider": Value Change {
        n227 = event-data() -> ("NewVal"=w357:dbl)  [unwired: 1 in]
        n228 = call <vilib>:"NT Write Number.vi"("Numeric"=w357, "Name"=w358) -> ()  [unwired: 9 in, 1 out]
      }
      event "On/Off": Value Change {
        n229 = event-data() -> ("NewVal"=w362:bool)  [unwired: 1 in]
        n230 = Boolean To (0,1)(Boolean=w362) -> (0, 1=w361:i16)
        n231 = call <vilib>:"NT Write Number.vi"("Numeric"=w361, "Name"=w360) -> ()  [unwired: 9 in, 1 out]
      }
      event "Rev/Fwd": Value Change {
        n232 = event-data() -> ("NewVal.Forward"=w370:bool, "NewVal.Reverse"=w369:bool)  [unwired: 1 in]
        n233 = Boolean To (0,1)(Boolean=w370) -> (0, 1=w366:i16)
        n234 = Boolean To (0,1)(Boolean=w369) -> (0, 1=w368:i16)
        n235 = Negate(x=w368) -> (-x=w367:i16)
        n236 = Add(x=w366, y=w367) -> (x+y=w365:i16)
        n237 = call <vilib>:"NT Write Number.vi"("Numeric"=w365, "Name"=w364) -> ()  [unwired: 9 in, 1 out]
      }
      event "Test Ring": Value Change {
        n238 = event-data() -> ("NewVal"=w374:u16)  [unwired: 1 in]
        n239 = property on="Test Ring" class="Ring (strict)"() -> ("Strings []"=w375:string[])  [unwired: 2 in, 2 out]
        n240 = Index Array(array=w375, index=w374) -> (element=w373:string)
        n241 = call <vilib>:"NT Write String.vi"("String"=w373, "Name"=w372) -> ()  [unwired: 9 in, 1 out]
      }
      event "Rec Mode": Value Change {
        # "Update globals for recording mode and path to read log from.\nClear when logging and let NetworkTables set path for vision to\nuse."
        n242 = event-data() -> ("NewVal"=w385:enum32{"Stop", "Record", "Playback"})  [unwired: 1 in]
        n243 = global write "WPI_DashboardLogging Global.vi" "Logging Filename"(path "") -> ()
        n244 = case shown="\"Stop\", \"Record\"" w385 {
          tunnel: w384 -> [_ w387 w395]
          tunnel: [_ _ w394] -> w381
          tunnel: [_ _ w393] -> _
          tunnel: w379 -> [_ _ w391]
          tunnel: cluster{i32, i32} {-250, 170} -> [_ _ w390]
          tunnel: [_ _ T11 {"Image Size"=TRUE, "Image Type"=TRUE, "Pixel Value"=TRUE, "ROI Information"=TRUE, "Zoom Factor"=FALSE} ("Image Information Shown:All Elements")] -> w377
          tunnel: [_ _ TRUE ("Zoom Factor")] -> w376
          frame Default {
          }
          frame "Stop", "Record" {
            # "Place Window too"
            n245 = invoke class="VI" method="FP.Close"(reference=w387) -> (reference out=w386:refnum<vi>)  [unwired: 2 in, 2 out]
            n246 = invoke class="VI" method="Abort VI"(reference=w386) -> ()  [unwired: 2 in, 3 out]
          }
          frame "Playback" {
            n247 = call "Open Playback Panel.vi"("Offset"=w390, "DB VI Ref"=w391, "Playback in"=w395) -> ("Playback out"=w392:refnum<vi>)  [unwired: 8 in]
            n248 = register-events(w392) -> (reference out=w394:refnum<event-registration>, error out=w393:errorcluster)  [unwired: 2 in]
          }
        }
        n249 = global write "WPI_DashboardLogging Global.vi" "Recording"(w385) -> ()
        n250 = property on="Camera Image" class="ImageControl"("Image Information Shown"=w377, "Image Information Visible"=w376) -> ()  [unwired: 2 in, 2 out]
        n251 = call <vilib>:"WPI_DashboardNT Log FieldName Cache.vi"("Operation"=enum16{"Lookup/Add", "Index", "Clear"}."Clear") -> ()  [unwired: 8 in, 3 out]
      }
      event Panel Close {
        w396 = enum32{"Stop", "Record", "Playback"}."Stop" ("Rec Mode")
        n252 = event-data() -> ()  [unwired: 1 in, 4 out]
        n253 = local write "Rec Mode"(w396) -> ()
        n254 = global write "WPI_DashboardLogging Global.vi" "Recording"(w396) -> ()
      }
      event Panel Close {
        # "Abort playback window and ourself"
        n255 = event-data() -> ()  [unwired: 1 in, 4 out]
        n256 = invoke class="VI" method="FP.Close"(reference=w401) -> (reference out=w400:refnum<vi>)  [unwired: 2 in, 2 out]
        n257 = invoke class="VI" method="Abort VI"(reference=w400) -> (error out=w399:errorcluster)  [unwired: 2 in, 2 out]
        n258 = invoke class="VI" method="Abort VI"(error in=w399) -> ()  [unwired: 2 in, 3 out]
      }
    }
  }
  n259 = property on="On/Off" class="Bool (strict)"("Visible"=w25) -> ()  [unwired: 2 in, 2 out]
  n260 = property on="Motor" class="Clust (strict)"("Visible"=w25) -> ()  [unwired: 2 in, 2 out]
  n261 = property on="Progress" class="Clust (strict)"("Visible"=w25) -> ()  [unwired: 2 in, 2 out]
  n262 = property on="Test Ring" class="Ring (strict)"("Visible"=w25) -> ()  [unwired: 2 in, 2 out]
  n263 = property on="Rev/Fwd" class="Clust (strict)"("Visible"=w25) -> ()  [unwired: 2 in, 2 out]
  n264 = property on="Camera Settings" class="Clust (strict)"("Visible"=w25) -> ()  [unwired: 2 in, 2 out]
  n265 = local write "DB Camera Config"(w25) -> ()
  n266 = global write "WPI_DashboardLogging Global.vi" "Recording"(w8) -> ()
  n267 = local write "Rec Mode"(w8) -> ()
